vi "Action Set Date & Time.vi"(0 "VISA resource name":refnum<visa-resource-name>, 1 "Hour (0)":dbl min=0.0 max=23.0 step=1.0, 2 "Minutes (0)":dbl min=0.0 max=59.0 step=1.0, 5 "Month (0: January)":u16(ring) items=["January", "February", "March", "April", "May", "June", "July", "August", "September", "October", "November", "December"], 7 "Day (1)":dbl=1.0 min=1.0 max=31.0 step=1.0, 9 "Year (1996)":dbl=1996.0 min=1996.0 max=9999.0 step=1.0, 11 "error in (no error)":errorcluster, 12 "Seconds (0)":dbl min=0.0 max=59.0 step=1.0, 13 "Milliseconds (0)":dbl min=0.0 max=999.0 step=10.0) -> (4 "VISA resource name out":refnum<visa-resource-name>, 15 "error out":errorcluster)   [LabVIEW 2020, in "Lake Shore Cryotronics 340.lvlib"]
doc: "This VI configures the date & time for the instrument using 24-hour format."
uses:
  Lake Shore Cryotronics 340.lvlib
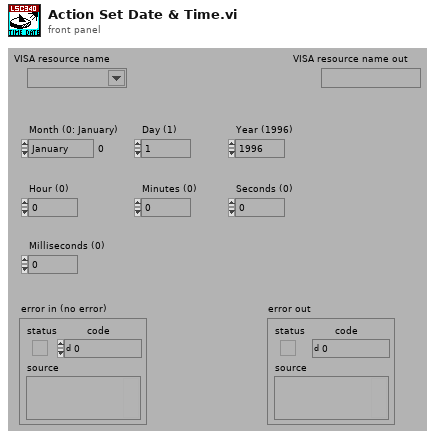
[diagram p1: front panel]
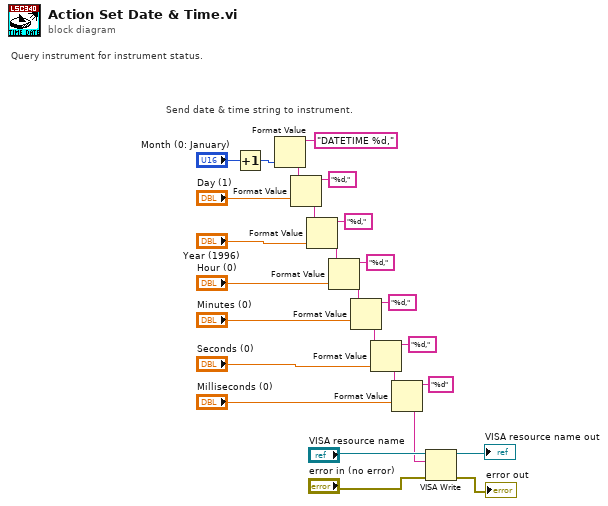
[diagram p0: block diagram]
diagram:
  # "Send date & time string to instrument."
  # "Query instrument for instrument status."
  n1 = Increment(x="Month (0: January)") -> (x+1=w6:u16)
  n2 = Format Value(format string="DATETIME %d,", value (0)=w6) -> (output string=w17:string)  [unwired: 1 in]
  n3 = Format Value(string ("")=w17, format string="%d,", value (0)="Day (1)") -> (output string=w16:string)
  n4 = Format Value(string ("")=w16, format string="%d,", value (0)="Year (1996)") -> (output string=w15:string)
  n5 = Format Value(string ("")=w15, format string="%d,", value (0)="Hour (0)") -> (output string=w14:string)
  n6 = Format Value(string ("")=w14, format string="%d,", value (0)="Minutes (0)") -> (output string=w12:string)
  n7 = Format Value(string ("")=w12, format string="%d,", value (0)="Seconds (0)") -> (output string=w13:string)
  n8 = Format Value(string ("")=w13, format string="%d", value (0)="Milliseconds (0)") -> (output string=w1:string)
  n9 = VISA Write(VISA resource name="VISA resource name", write buffer=w1, error in (no error)="error in (no error)") -> (VISA resource name out=→"VISA resource name out":refnum<visa-resource-name>, error out=→"error out":errorcluster)  [unwired: 1 out]
